vi "get single spec.vi"(10 "single item name":string, 11 "single spec":T1={"limit Spec"=array1616x8[12928 elements], "Diff Test Item Name"=["SDD21", "SDD11", "SCD22", "SCC11", "SCD21-SDD21", "NEXT", "ILD_15"], "Spec _Col"=[1, 2, 3, 4, 5, 6, 7]}) -> (3 "single spec":dbl[](array[numeric]))   [LabVIEW 2011]
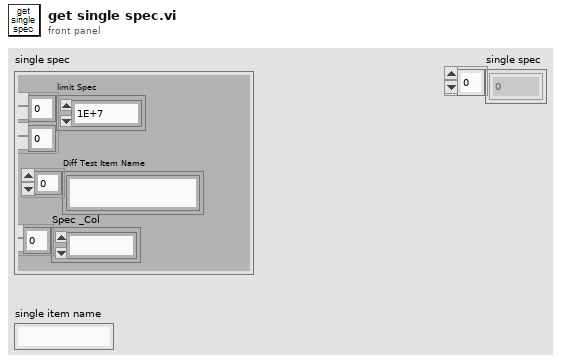
[diagram p1: front panel]
types:
  T1 = cluster{"limit Spec":dbl[][], "Diff Test Item Name":string[], "Spec _Col":i32[]}
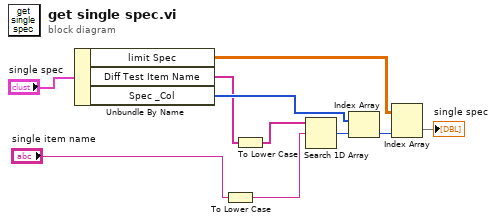
[diagram p0: block diagram]
diagram:
  n1 = Unbundle By Name("single spec") -> ("limit Spec"=w7:dbl[][], "Diff Test Item Name"=w4:string[], "Spec _Col"=w9:i32[])
  n2 = To Lower Case(string="single item name") -> (all lower case string=w1:string)
  n3 = To Lower Case(string=w4) -> (all lower case string=w3:string[])
  n4 = Search 1D Array(1D array=w3, element=w1) -> (index of element=w8:i32)  [unwired: 1 in]
  n5 = Index Array(array=w9, index=w8) -> (element=w6:i32)
  n6 = Index Array(array=w7, index (col)=w6) -> (element=→"single spec":dbl[])  [unwired: 1 in]
